vi "Initialize.vi"(8 "ErrorIn":errorcluster, 10 "Modul Type to Simulate":T2 items=["Hardware Modus"=0, "SPC-600 Simulation"=600, "SPC-630 Simulation"=630, "SPC-700  Simulation"=700, "SPC-730  Simulation"=730, "SPC-130  Simulation"=130, "SPC-830  Simulation"=830, "SPC-140  Simulation"=140, "SPC-930  Simulation"=930, "DPC-230  Simulation"=230, "SPC-150  Simulation"=150, "SPC-150 N  Simulation"=151, "SPC-150 NX  Simulation"=152, "SPC-130 EM  Simulation"=131, "SPC-130 EMN  Simulation"=132, "SPC-130 IN Simulation"=135, "SPC-130 INX Simulation"=136, "SPC-130 INXX Simulation"=137, "SPC-160  Simulation"=160, "SPC-160 X  Simulation"=161, "SPC-160 PCIE  Simulation"=162, "SPC-180 Simulation"=180, "SPC-181 Simulation"=181, "SPC-182 Simulation"=182, "SPC-185 Simulation"=185, "SPC-186 Simulation"=186, "SPC-187 Simulation"=187, "DPC-330  Simulation"=330, "DPC-590  Simulation"=590, "TDC-104 Simulation"=104], 11 "Init Cluster":T1) -> (0 "ErrorOut":errorcluster, 1 "SerialNumbersArray":string[](array[string]), 2 "ModuleNoArray":i16[](array[numeric]), 3 "DLL Path":path, 5 "SPCModulesArray":T3[](array[typedef]) {"Bus Number" min=-1 max=255 step=1; "Base I/O Addr" format="%.0x"; "Init Status" min=-10 max=0 step=1; "in Use" min=-1 max=1 step=1; "Slot Number" min=-1 max=255 step=1; "Module Type" items=["SPC-600"=600, "SPC-630"=630, "SPC-700"=700, "SPC-730"=730, "SPC-130"=130, "SPC-830"=830, "SPC-140"=140, "SPC-930"=930, "DPC-230"=230, "SPC-150"=150, "SPC-150 N"=151, "SPC-150 NX"=152, "SPC-130 EM"=131, "SPC-130 EMN"=132, "SPC-160"=160, "SPC-160 X"=161, "SPC-160 PCIE"=162, "SPC-180 N"=180, "SPC-180 NX"=181, "SPC-180 NXX"=182, "SPC-180 N-USB"=185, "SPC-180 NX-USB"=186, "SPC-180 NXX-USB"=187, "TDC-104"=104, "DPC-330"=330, "SPC-590"=590, "Simulation"=-1]})   [LabVIEW 2019]
doc: "This is a convenience VI combining several spcmdll calls all needed to successfully initialize communication to SPC modules.\nBefore a measurement is started the measurement parameter values must be written into the internal structures of the DLL functions (not directly visible from the user program) and sent to the control registers of the SPC module(s). This is accomplished by the function SPC_init. The function\n- checks whether DLL is correctly registered ( looks for a BH license number and verifies it)\n- reads the parameter values from the specified file ini_file\n- checks and recalculates the parameters depending on hardware restrictions and adjust parameters from the EEPROM on the SPC module(s)\n- sends the parameter values to the internal structures of the DLL \n- sends the parameter values to the SPC control registers\n- performs a hardware test of the SPC module(s)\nThe module will be initialised, but only when it is not in use (locked) by other application.\nAfter successful initialisation the module is locked to prevent that other application can access it. The user should check initialisation status of all modules he wants to use by calling SPC_get_init_status function.\nIf, for some reasons, the module which was locked must be initialised, it can be done using the function SPC_set_mode with the parameter 'force_use' = 1. \nThe initialisation file is an ASCII file with a structure shown in the table below. We recommend either to use the file spcm.ini or to start with spcm.ini and introduce the desired changes.\n\ninfo@becker-hickl.com"
uses:
  SPC_Controls/SPCModInfo.ctl
  SPC_Controls/ModuleType.ctl
  SPC_Controls/ModuleTypes.ctl
  SPC_Controls/InitCluster.ctl
panel:
  out "Number of Usable Modules":i16 min=0 max=8
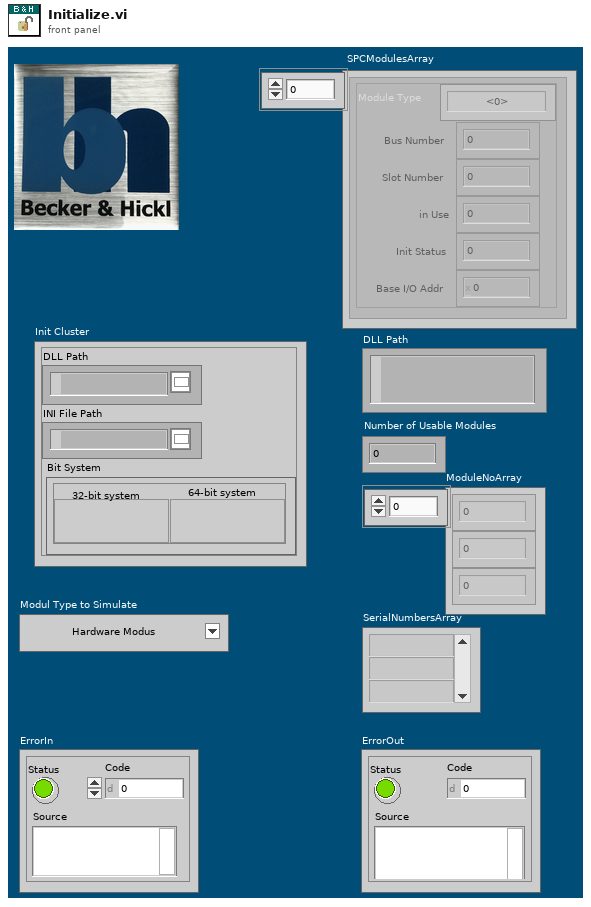
[diagram p1: front panel]
types:
  T1 = typedef "InitCluster.ctl" = cluster{"DLL Path":path, "INI File Path":path, "Bit System":cluster{"32-bit system":bool, "64-bit system":bool}}
  T2 = typedef "ModuleTypes.ctl" = i16
  T3 = typedef "SPCModInfo.ctl" = cluster{"Module Type":T4, "Bus Number":i16, "Slot Number":i16, "in Use":i16, "Init Status":i16, "Base I/O Addr":u16}
  T4 = typedef "ModuleType.ctl" = i16
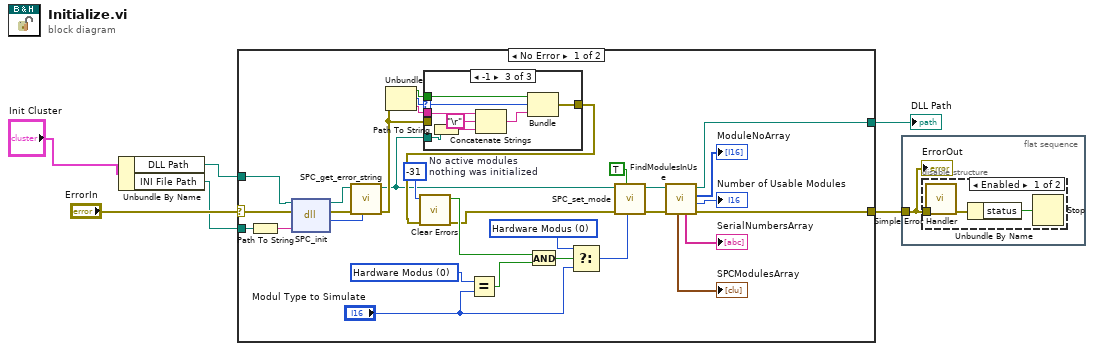
[diagram p0: block diagram]
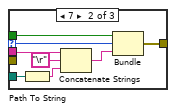
[diagram p4: hidden frame]
diagram:
  n1 = Unbundle By Name("Init Cluster") -> ("DLL Path"=w3:path, "INI File Path"=w2:path)
  n2 = case shown="No Error" "ErrorIn" {
    selector: "ErrorIn" -> [w25 w56]
    tunnel: [w37 w55] -> w6
    tunnel: [w36 w56] -> w5
    tunnel: w3 -> [w8 w55]
    tunnel: w2 -> [w7 _]
    frame No Error {
      w18 = T2 0 items=["Hardware Modus"=0, "SPC-600 Simulation"=600, "SPC-630 Simulation"=630, "SPC-700  Simulation"=700, "SPC-730  Simulation"=730, "SPC-130  Simulation"=130, "SPC-830  Simulation"=830, "SPC-140  Simulation"=140, "SPC-930  Simulation"=930, "DPC-230  Simulation"=230, "SPC-150  Simulation"=150, "SPC-150 N  Simulation"=151, "SPC-150 NX  Simulation"=152, "SPC-130 EM  Simulation"=131, "SPC-130 EMN  Simulation"=132, "SPC-160  Simulation"=160, "SPC-160 X  Simulation"=161, "SPC-160 PCIE  Simulation"=162, "DPC-330  Simulation"=330, "DPC 590  Simulation"=590] ("x")
      w22 = T2 0 items=["Hardware Modus"=0, "SPC-600 Simulation"=600, "SPC-630 Simulation"=630, "SPC-700  Simulation"=700, "SPC-730  Simulation"=730, "SPC-130  Simulation"=130, "SPC-830  Simulation"=830, "SPC-140  Simulation"=140, "SPC-930  Simulation"=930, "DPC-230  Simulation"=230, "SPC-150  Simulation"=150, "SPC-150 N  Simulation"=151, "SPC-150 NX  Simulation"=152, "SPC-130 EM  Simulation"=131, "SPC-130 EMN  Simulation"=132, "SPC-160  Simulation"=160, "SPC-160 X  Simulation"=161, "SPC-160 PCIE  Simulation"=162, "DPC-330  Simulation"=330, "DPC 590  Simulation"=590] ("t")
      w23 = -31  # No active modules nothing was initialized
      n3 = Path To String(path=w7) -> (string=w26:string)
      n4 = dll-call lib="D:/spcm/lib/lab_view/lv10.0/spcm32.dll" fn="SPC_init"(path in=w8, error in=w25, "ini_file"=w26) -> (path out=w27:path, error out=w29:errorcluster, "return type"=w28:i16)  [unwired: 2 in]
      n5 = call "SPC_get_error_string.vi"("ErrorID"=w28, "Error In"=w29, "DLL Path"=w27) -> ("Error Out"=w12:errorcluster, "DLL Path"=w11:path)  [unwired: 6 in, 1 out]
      n6 = Unbundle(w12) -> ("Status"=w14:bool, "Code"=w16:i32, "Source"=w15:string)
      n7 = case shown="-1" w16 {
        selector: w16 -> [_ w41 w50]
        tunnel: w15 -> [_ w46 w54]
        tunnel: w11 -> [_ w45 w47]
        tunnel: w14 -> [_ w40 w49]
        tunnel: [w38 w39 w48] -> w13
        tunnel: w12 -> [w38 _ _]
        frame Default {
        }
        frame 7 {
          n8 = Path To String(path=w45) -> (string=w44:string)
          n9 = Concatenate Strings(w46, "\r", w44) -> (w42:string)
          n10 = Bundle("Status"=w40, "Code"=w41, w42) -> (w39:cluster{"Status":bool, "Code":i32, string})  [unwired: 1 in]
        }
        frame -1 {
          n11 = Path To String(path=w47) -> (string=w53:string)
          n12 = Concatenate Strings(w54, "\r", w53) -> (w51:string)
          n13 = Bundle("Status"=w49, "Code"=w50, w51) -> (w48:cluster{"Status":bool, "Code":i32, string})  [unwired: 1 in]
        }
      }
      n14 = call <vilib>:"Clear Errors.vi"("error in (no error)"=w13, "specific error code to clear (0: all)"=w23) -> ("error out"=w9:errorcluster, "specific error cleared?"=w21:bool)  [unwired: 4 in]
      n15 = Equal?(x=w18, y="Modul Type to Simulate") -> (x = y?=w17:bool)
      n16 = And(x=w21, y=w17) -> (x .and. y?=w20:bool)
      n17 = Select(t=w22, s=w20, f="Modul Type to Simulate") -> (s? t:f=w24:T2)
      n18 = call "SPC_set_mode.vi"("Modul Type to Simulate"=w24, "Force Use"=TRUE, "Error In"=w9, "DLL Path"=w11) -> ("Error Out"=w30:errorcluster, "DLL Path"=w31:path)  [unwired: 6 in]
      n19 = call "FindModulesInUse.vi"("Error In"=w30, "DLL Path"=w31) -> ("Error Out"=w36:errorcluster, "Number of Usable Modules"=→"Number of Usable Modules":i16, "ModuleNoArray"=→"ModuleNoArray":i16[], "DLL Path"=w37:path, "Array Of Serialnumbers"=→"SerialNumbersArray":string[], "SPCModulesArray"=→"SPCModulesArray":T3[])  [unwired: 4 in]
    }
    frame Error {
    }
  }
  "DLL Path" <- w6
  n20 = flat-sequence {
    tunnel: w5 -> [w57]
    frame #0 {
      n21 = disable-structure shown="Enabled" {
        disable-tunnel: w57 -> [w59 _]
        frame Enabled {
          n22 = call <vilib>:"Simple Error Handler.vi"("error in (no error)"=w59) -> ("error out"=w58:errorcluster)  [unwired: 4 in, 4 out]
          n23 = Unbundle By Name(w58) -> ("status"=w60:bool)
          n24 = Stop(stop? (T)=w60) -> ()
        }
        frame Disabled {
        }
      }
      "ErrorOut" <- w57
    }
  }
